vi "CRYUpdate Controls.vi"() -> (0 "Unprotect?":bool, 1 "Protect?":bool, 2 "Delete/Rename?":bool, 3 "Save/Export?":bool, 4 "AutoProtect?":bool, 5 "Import?":bool, 6 "UndoAutoProtect?":bool)   [LabVIEW 2013]
uses:
  CRYMainGlobal.vi
panel:
  # "Update Various Controls"
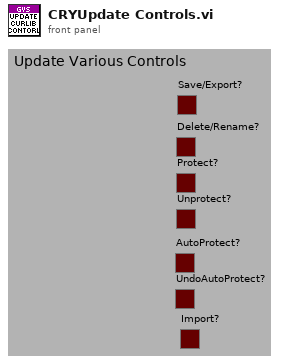
[diagram p1: front panel]
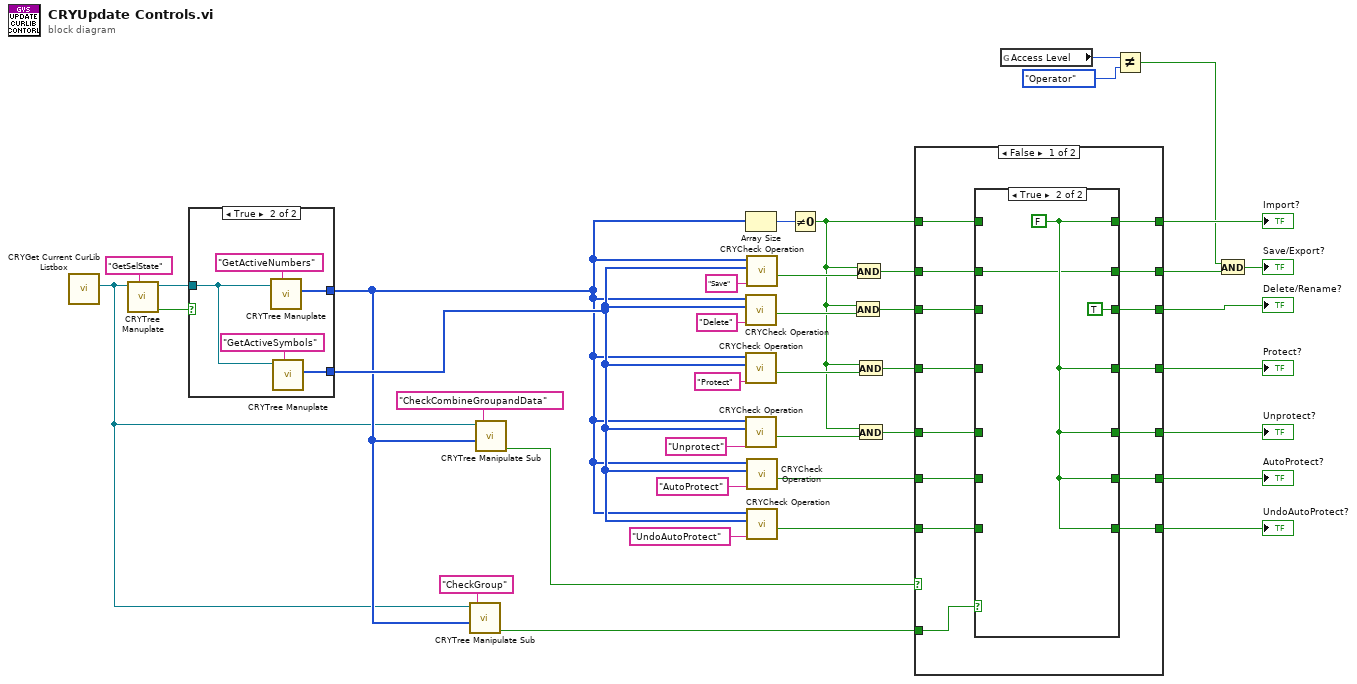
[diagram p0: block diagram]
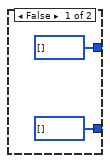
[diagram p2: hidden frame]
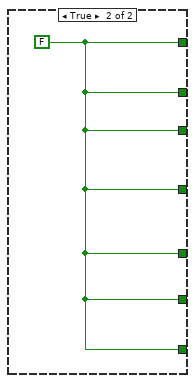
[diagram p4: hidden frame]
diagram:
  n1 = call "CRYGet Current CurLib Listbox.vi"() -> ("CurLib Tree"=w7:refnum<vi>)  [unwired: 9 in, 2 out]
  n2 = call "CRYTree Manuplate.vi"("sAction"="GetSelState", "Tree in"=w7) -> ("bResult Out"=w13:bool, "Tree Out"=w12:refnum<vi>)  [unwired: 6 in, 2 out]
  n3 = case shown="True" w13 {
    tunnel: [i32[] [] ("nData Out") w44] -> w8
    tunnel: [i32[] [] ("nData Out") w43] -> w11
    tunnel: w12 -> [_ w42]
    frame False {
    }
    frame True {
      n4 = call "CRYTree Manuplate.vi"("sAction"="GetActiveNumbers", "Tree in"=w42) -> ("nData Out"=w44:i32[])  [unwired: 6 in, 3 out]
      n5 = call "CRYTree Manuplate.vi"("sAction"="GetActiveSymbols", "Tree in"=w42) -> ("nData Out"=w43:i32[])  [unwired: 6 in, 3 out]
    }
  }
  n6 = call "CRYTree Manipulate Sub.vi"("sAction"="CheckGroup", "nData"=w8, "Tree in"=w7) -> ("bData out"=w9:bool)  [unwired: 4 in, 4 out]
  n7 = call "CRYTree Manipulate Sub.vi"("sAction"="CheckCombineGroupandData", "nData"=w8, "Tree in"=w7) -> ("bData out"=w10:bool)  [unwired: 4 in, 4 out]
  n8 = Array Size(array=w8) -> (size(s)=w39:i32)
  n9 = call "CRYCheck Operation.vi"("Operation"="Delete", "Item Symbols In"=w11, "Index Array In"=w8) -> ("Operation ?"=w38:bool)  [unwired: 1 in, 7 out]
  n10 = call "CRYCheck Operation.vi"("Operation"="Protect", "Item Symbols In"=w11, "Index Array In"=w8) -> ("Operation ?"=w37:bool)  [unwired: 6 in, 2 out]
  n11 = call "CRYCheck Operation.vi"("Operation"="Unprotect", "Item Symbols In"=w11, "Index Array In"=w8) -> ("Operation ?"=w36:bool)  [unwired: 6 in, 2 out]
  n12 = call "CRYCheck Operation.vi"("Operation"="Save", "Item Symbols In"=w11, "Index Array In"=w8) -> ("Operation ?"=w29:bool)  [unwired: 1 in, 7 out]
  n13 = call "CRYCheck Operation.vi"("Operation"="AutoProtect", "Item Symbols In"=w11, "Index Array In"=w8) -> ("Operation ?"=w22:bool)  [unwired: 6 in, 2 out]
  n14 = call "CRYCheck Operation.vi"("Operation"="UndoAutoProtect", "Item Symbols In"=w11, "Index Array In"=w8) -> ("Operation ?"=w21:bool)  [unwired: 6 in, 2 out]
  n15 = Not Equal To 0?(x=w39) -> (x != 0?=w16:bool)
  n16 = And(x=w16, y=w38) -> (x .and. y?=w25:bool)
  n17 = And(x=w16, y=w29) -> (x .and. y?=w26:bool)
  n18 = And(x=w16, y=w37) -> (x .and. y?=w24:bool)
  n19 = And(x=w16, y=w36) -> (x .and. y?=w23:bool)
  n20 = case shown="False" w10 {
    tunnel: [w58 w72] -> w4
    tunnel: w26 -> [w59 _]
    tunnel: w25 -> [w57 _]
    tunnel: [w56 w72] -> w1
    tunnel: w24 -> [w55 _]
    tunnel: [w54 w72] -> w17
    tunnel: w23 -> [w53 _]
    tunnel: [w52 w72] -> w18
    tunnel: w22 -> [w51 _]
    tunnel: [w50 w72] -> w19
    tunnel: w21 -> [w49 _]
    tunnel: [w48 w72] -> w20
    tunnel: w16 -> [w61 _]
    tunnel: [w60 w72] -> w15
    tunnel: w9 -> [w47 _]
    frame False {
      n21 = case shown="True" w47 {
        tunnel: w61 -> [w68 _]
        tunnel: [w68 w71] -> w60
        tunnel: w59 -> [w67 w70]
        tunnel: [w67 w70] -> w58
        tunnel: w57 -> [w66 _]
        tunnel: [w66 TRUE] -> w56
        tunnel: w55 -> [w65 _]
        tunnel: [w65 w71] -> w54
        tunnel: w53 -> [w64 _]
        tunnel: [w64 w71] -> w52
        tunnel: w51 -> [w63 _]
        tunnel: [w63 w71] -> w50
        tunnel: w49 -> [w62 _]
        tunnel: [w62 w71] -> w48
        frame False {
        }
        frame True {
          w71 = FALSE
        }
      }
    }
    frame True {
      w72 = FALSE
    }
  }
  "Delete/Rename?" <- w1
  "Protect?" <- w17
  "Unprotect?" <- w18
  "AutoProtect?" <- w19
  "UndoAutoProtect?" <- w20
  "Import?" <- w15
  n22 = global read "CRYMainGlobal.vi" "Access Level"() -> (w6:enum16{"Engineer", "Technician", "Operator"})
  n23 = Not Equal?(x=w6, y=enum16{"Engineer", "Technician", "Operator"}."Operator") -> (x != y?=w2:bool)
  n24 = And(x=w2, y=w4) -> (x .and. y?=→"Save/Export?":bool)
